vi "Axis Array Constants.vi"(11 "Numeric":i32) -> (3 "Axis Constants":refnum<k21>[](array[refnum]))   [LabVIEW 2015]
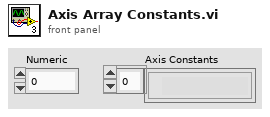
[diagram p1: front panel]
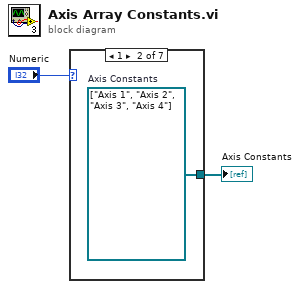
[diagram p0: block diagram]
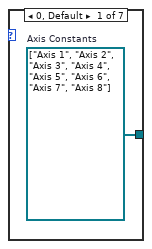
[diagram p2: hidden frame]
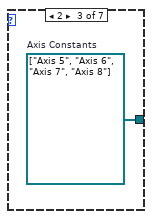
[diagram p3: hidden frame]
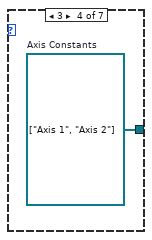
[diagram p4: hidden frame]
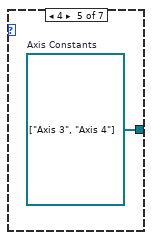
[diagram p5: hidden frame]
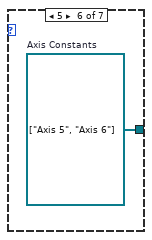
[diagram p6: hidden frame]
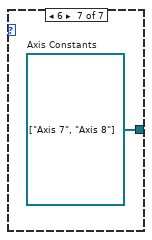
[diagram p7: hidden frame]
diagram:
  n1 = case shown="1" "Numeric" {
    tunnel: [w3 w4 w5 w6 w7 w8 w9] -> w1
    frame 0, Default {
      w3 = refnum<k21>[] ["Axis 1", "Axis 2", "Axis 3", "Axis 4", "Axis 5", "Axis 6", "Axis 7", "Axis 8"]  # Axis Constants
    }
    frame 1 {
      w4 = refnum<k21>[] ["Axis 1", "Axis 2", "Axis 3", "Axis 4"]  # Axis Constants
    }
    frame 2 {
      w5 = refnum<k21>[] ["Axis 5", "Axis 6", "Axis 7", "Axis 8"]  # Axis Constants
    }
    frame 3 {
      w6 = refnum<k21>[] ["Axis 1", "Axis 2"]  # Axis Constants
    }
    frame 4 {
      w7 = refnum<k21>[] ["Axis 3", "Axis 4"]  # Axis Constants
    }
    frame 5 {
      w8 = refnum<k21>[] ["Axis 5", "Axis 6"]  # Axis Constants
    }
    frame 6 {
      w9 = refnum<k21>[] ["Axis 7", "Axis 8"]  # Axis Constants
    }
  }
  "Axis Constants" <- w1
